vi "Query All Types.vi"(6 "timeout (ms)":i32=5000, 8 "error in":errorcluster, 10 "reload":bool, 11 "gRPC ID in":T4) -> (0 "error out":errorcluster, 2 "plugin_types":T1[](array[typedef]), 3 "gRPC ID out":T4)   [LabVIEW 2021, in "CIFManagerClientWrapper.lvlib"]
uses:
  CIFManagerClientWrapper.lvlib
  <vilib>/gRPC/LabVIEW gRPC Library/Shared/grpcId.ctl
  CIF_Manager_client/RPC Messages/cif_manager_PluginType.ctl
  CIF_Manager_client/RPC Messages/cif_common_ShortVersion.ctl
  CIF_Manager_client/RPC Messages/cif_management_common_PluginMetadata.ctl
  CIF_Manager_client/RPC Messages/cif_manager_QueryPluginTypesRequest.ctl
  CIF_Manager_client/CIF_Manager_client.lvlib
  <vilib>/gRPC/LabVIEW gRPC Library/grpc-lvsupport-release.lvlib
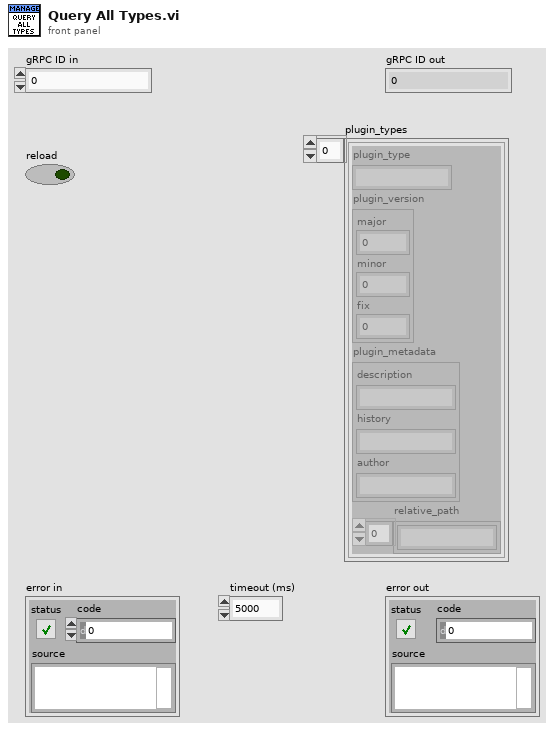
[diagram p1: front panel]
types:
  T1 = typedef "CIF_Manager_client.lvlib/cif_manager_PluginType.ctl" = cluster{"plugin_type":string, "plugin_version":T2, "plugin_metadata":T3, "relative_path":string[]}
  T2 = typedef "CIF_Manager_client.lvlib/cif_common_ShortVersion.ctl" = cluster{"major":u32, "minor":u32, "fix":u32}
  T3 = typedef "CIF_Manager_client.lvlib/cif_management_common_PluginMetadata.ctl" = cluster{"description":string, "history":string, "author":string}
  T4 = typedef "grpc-lvsupport-release.lvlib/grpcId.ctl" = u64
  T5 = typedef "CIF_Manager_client.lvlib/cif_manager_QueryPluginTypesRequest.ctl" = cluster{"reload":bool}
  T6 = typedef "CIF_Manager_client.lvlib/cif_manager_QueryPluginTypesResponse.ctl" = cluster{"plugin_types":T1[]}
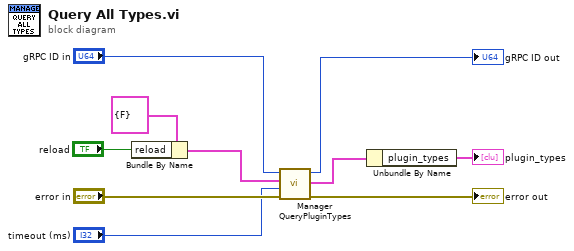
[diagram p0: block diagram]
diagram:
  n1 = Bundle By Name(cluster=T5 {"reload"=FALSE} ("Request Data"), "reload"="reload") -> (w2:T5)
  n2 = call "Manager QueryPluginTypes.vi"("error in"="error in", "timeout (ms)"="timeout (ms)", "Request Data"=w2, "gRPC ID"="gRPC ID in") -> ("error out"=→"error out":errorcluster, "Response Data"=w6:T6, "gRPC ID out"=→"gRPC ID out":T4)  [unwired: 5 in]
  n3 = Unbundle By Name(w6) -> ("plugin_types"=→"plugin_types":T1[])
